vi "LoggerConvertDetailEnumToString.vi"(5 "Log Type":enum16{"Debug", "Info", "Error", "Warn"}(ring)) -> (2 "String":string)   [LabVIEW 2014]
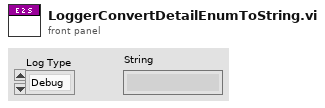
[diagram p1: front panel]
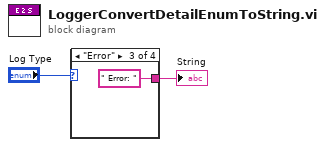
[diagram p0: block diagram]
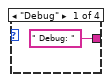
[diagram p2: hidden frame]
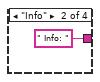
[diagram p3: hidden frame]
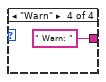
[diagram p4: hidden frame]
diagram:
  n1 = case shown="\"Error\"" "Log Type" {
    tunnel: [" Debug: " " Info: " " Error: " " Warn: "] -> w1
    frame "Debug" {
    }
    frame "Info" {
    }
    frame "Error" {
    }
    frame "Warn" {
    }
  }
  "String" <- w1
